vi "Projeto PI.vi"() -> ()   [LabVIEW 2020]
uses:
  <vilib>/Instr/_visa.llb/VISA Configure Serial Port (Instr).vi
panel:
  out "Direção (º)":i32(knob) scale=0.0..315.0
  out "M/S":i32(knob) scale=0.0..50.0
  out "KM/H":i32(knob) scale=0.0..50.0
  out "RPM":i32(knob) scale=0.0..1000.0
  out "Umidade":i32(slide) scale=0.0..100.0
  out "Temperatura":i32(slide) scale=0.0..50.0
  in  "stop":bool
  in  "VISA resource name":refnum<visa-resource-name>
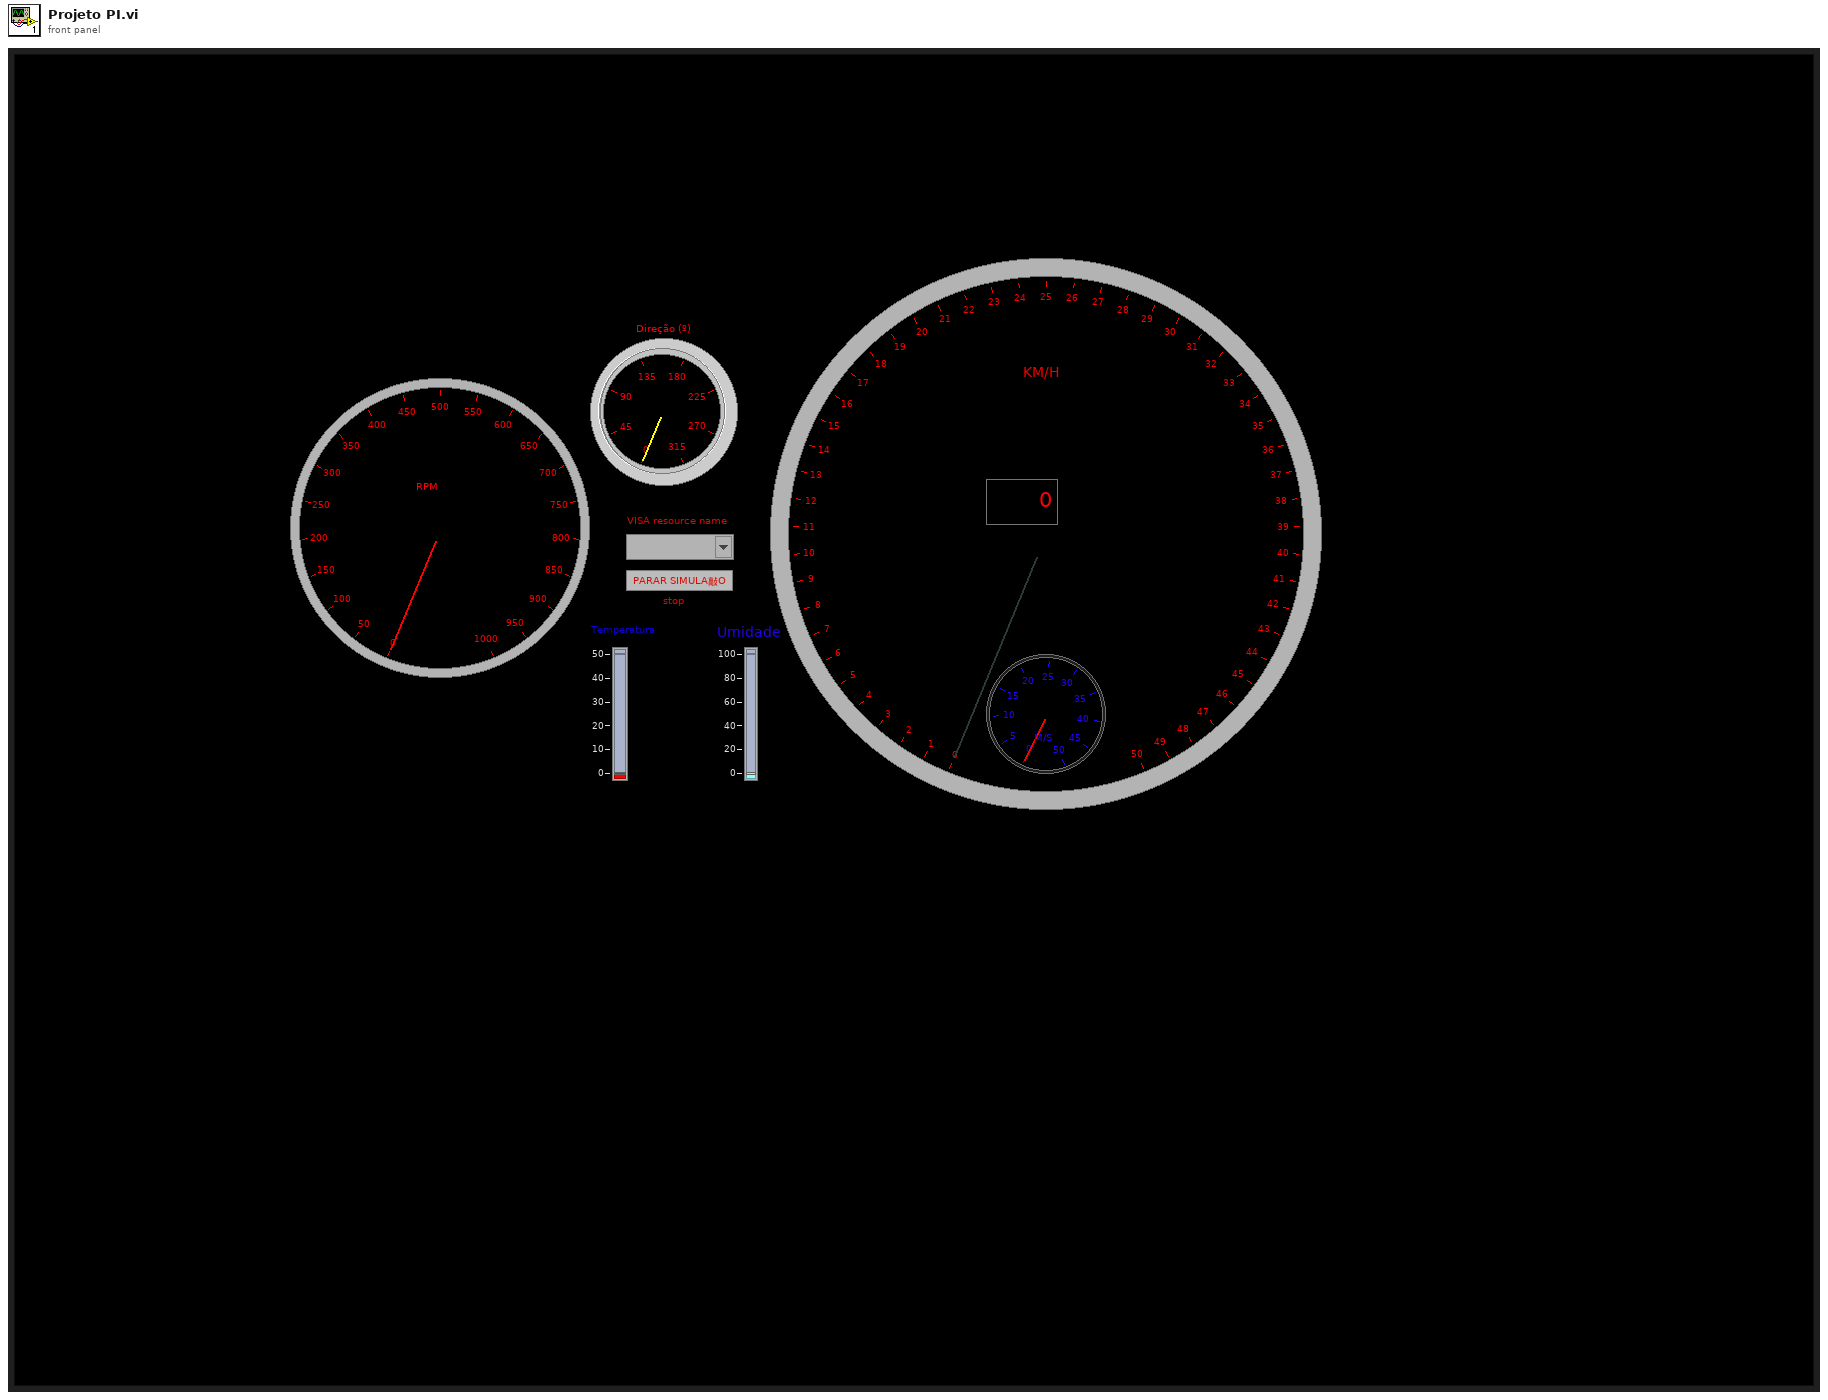
[diagram p1: front panel]
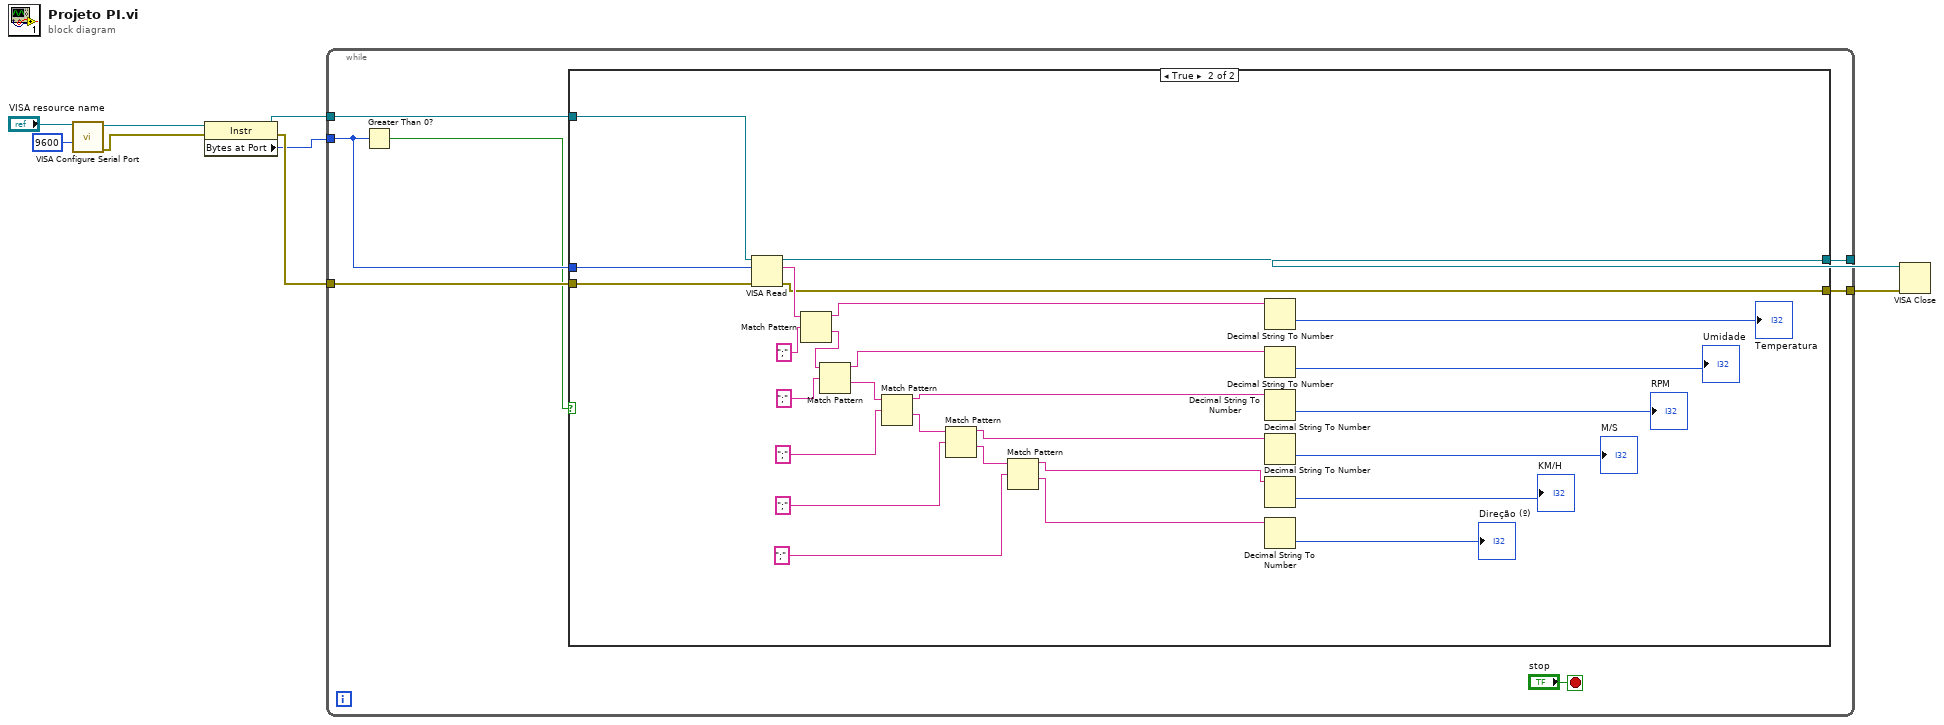
[diagram p0: block diagram]
diagram:
  n1 = call-poly "VISA Configure Serial Port"("VISA resource name"="VISA resource name", "baud rate (9600)"=u32 9600) -> ("VISA resource name out"=w9:refnum<visa-resource-name>, "error out"=w2:errorcluster)  [unwired: 12 in]
  n2 = property class="Instr"(reference=w9, error in=w2) -> (reference out=w1:refnum<visa-resource-name>, error out=w8:errorcluster, "Bytes at Port"=w7:u32)
  n3 = while {
    tunnel: w7 -> [w11]
    tunnel: w8 -> [w15]
    tunnel: [w13] -> w6
    tunnel: [w14] -> w5
    tunnel: w1 -> [w12]
    stop <- "stop" stop-if-true
    n4 = Greater Than 0?(x=w11) -> (x > 0?=w10:bool)
    n5 = case shown="True" w10 {
      tunnel: w15 -> [w17 w41]
      tunnel: [w18 w45] -> w13
      tunnel: [w17 w42] -> w14
      tunnel: w12 -> [w18 w22]
      tunnel: w11 -> [_ w21]
      frame False {
      }
      frame True {
        n6 = VISA Read(VISA resource name=w22, byte count=w21, error in (no error)=w41) -> (VISA resource name out=w45:refnum<visa-resource-name>, read buffer=w43:string, error out=w42:errorcluster)  [unwired: 1 out]
        n7 = Match Pattern(string=w43, regular expression=";") -> (before substring=w37:string, after substring=w20:string)  [unwired: 1 in, 2 out]
        n8 = Match Pattern(string=w20, regular expression=";") -> (before substring=w36:string, after substring=w40:string)  [unwired: 1 in, 2 out]
        n9 = Match Pattern(string=w40, regular expression=";") -> (before substring=w35:string, after substring=w39:string)  [unwired: 1 in, 2 out]
        n10 = Match Pattern(string=w39, regular expression=";") -> (before substring=w34:string, after substring=w38:string)  [unwired: 1 in, 2 out]
        n11 = Match Pattern(string=w38, regular expression=";") -> (before substring=w27:string, after substring=w28:string)  [unwired: 1 in, 2 out]
        n12 = Decimal String To Number(string=w37) -> (number=→"Temperatura":i32)  [unwired: 2 in, 1 out]
        n13 = Decimal String To Number(string=w36) -> (number=→"Umidade":i32)  [unwired: 2 in, 1 out]
        n14 = Decimal String To Number(string=w35) -> (number=→"RPM":i32)  [unwired: 2 in, 1 out]
        n15 = Decimal String To Number(string=w34) -> (number=→"M/S":i32)  [unwired: 2 in, 1 out]
        n16 = Decimal String To Number(string=w27) -> (number=→"KM/H":i32)  [unwired: 2 in, 1 out]
        n17 = Decimal String To Number(string=w28) -> (number=→"Direção (º)":i32)  [unwired: 2 in, 1 out]
      }
    }
  }
  n18 = VISA Close(VISA resource name=w6, error in (no error)=w5) -> ()  [unwired: 1 out]
